vi "passIf.vi"(7 "custom report message (\"\")":string, 8 "error in (no error)":errorcluster, 9 "message (\"\")":string, 10 "pass":bool, 11 "TestCase in":refnum<class "TestCase.lvclass">) -> (0 "error out":errorcluster, 3 "TestCase out":refnum<class "TestCase.lvclass">)   [LabVIEW 2013, in "TestCase.lvclass"]
doc: "Pass if 'pass' condition is TRUE. On failure, 'message' is appended to failure status."
uses:
  TestCase.lvclass
  TestCase.lvclass/TestCase.ctl
panel:
  # "JKI VI Tester for LabVIEW\nhttp://jkisoft.com/vi-tester\nCopyright (C) 2007-2009, JKI <info@jkisoft.com>\nALL RIGHTS RESERVED"
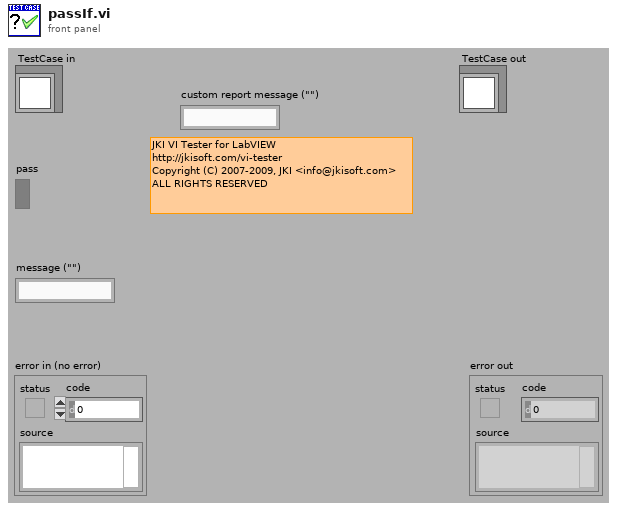
[diagram p1: front panel]
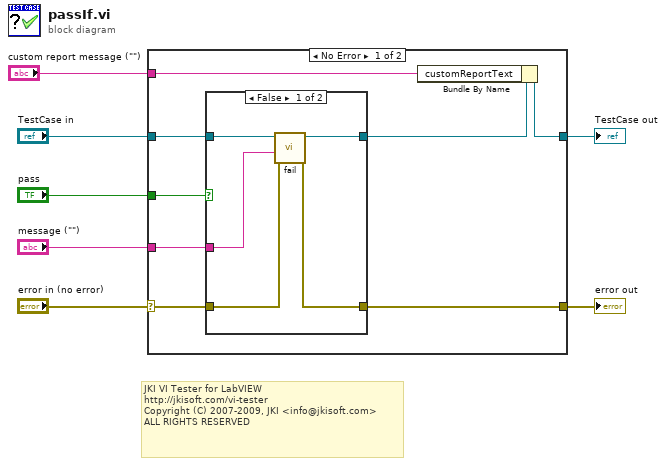
[diagram p0: block diagram]
diagram:
  # "JKI VI Tester for LabVIEW\nhttp://jkisoft.com/vi-tester\nCopyright (C) 2007-2009, JKI <info@jkisoft.com>\nALL RIGHTS RESERVED"
  n1 = case shown="No Error" "error in (no error)" {
    selector: "error in (no error)" -> [w15 w24]
    tunnel: [w14 w24] -> w3
    tunnel: [w9 w23] -> w4
    tunnel: "TestCase in" -> [w11 w23]
    tunnel: "message (\"\")" -> [w13 _]
    tunnel: "pass" -> [w12 _]
    tunnel: "custom report message (\"\")" -> [w8 _]
    frame No Error {
      n2 = case shown="False" w12 {
        tunnel: w15 -> [w20 w22]
        tunnel: [w19 w22] -> w14
        tunnel: w13 -> [w18 _]
        tunnel: w11 -> [w17 w21]
        tunnel: [w16 w21] -> w10
        frame False {
          n3 = call-dynamic "fail.vi"("error in (no error)"=w20, "message (\"\")"=w18, "TestCase in"=w17) -> ("error out"=w19:errorcluster, "TestCase out"=w16:refnum<class "TestCase.lvclass">)  [unwired: 7 in]
        }
        frame True {
        }
      }
      n4 = Bundle By Name(cluster=w10, "customReportText"=w8) -> (w9:refnum<class "TestCase.lvclass">)
    }
    frame Error {
    }
  }
  "error out" <- w3
  "TestCase out" <- w4
